vi "Test - Point At.vi"() -> ()   [LabVIEW 2020, in "3D.lvlib"]
uses:
  Vector 3D.ctl
  3D.lvlib
panel:
  out "Point At Matrix":sgl[][](array[numeric])
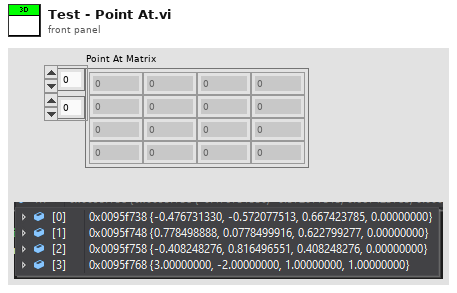
[diagram p1: front panel]
types:
  T1 = typedef "3D.lvlib/Vector 3D.ctl" = cluster{"x":sgl, "y":sgl, "z":sgl}
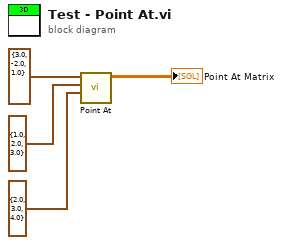
[diagram p0: block diagram]
diagram:
  n1 = call "Point At.vi"("Up"=T1 {"x"=2.0, "y"=3.0, "z"=4.0}, "Target"=T1 {"x"=1.0, "y"=2.0, "z"=3.0}, "Position"=T1 {"x"=3.0, "y"=-2.0, "z"=1.0}) -> ("Point At Matrix"=→"Point At Matrix":sgl[][])  [unwired: 8 in]
